vi "qEAX.vi"(0 "System no.":i32=1 min=1 max=4 step=1, 2 "Axes to query":string[](array[string]), 3 "All axes?":bool, 4 "Axis identifier?":bool=TRUE, 5 "error in":errorcluster) -> (14 "Axes enabled status":bool[](array[boolean]), 19 "error out":errorcluster)   [LabVIEW 2026]
doc: "GCS 3.0\n=====\n\nEAX? (Get Axis Activation State)\n\nDescription\nQueries the activation state of the axes.\nThe activation state of an axis corresponds to the switch-on state of its drive.\n\nFormat\nEAX?[ <AxisID>]\n\nArguments\nEAX? without arguments queries all axes of the controller.\n<AxisID>\nAn axis of the controller\nThe available axes can be queried with USG? SYS.\nPossible values: Alias of the axis\n\nResponse\n{<AxisID>\"=\"<ActivationState>LF}\n<ActivationState>\nActivation state of the axis\nCorresponds to the switch-on state of the drive of the axis\nPossible values:\n0 = Axis deactivated = Drive switched off\n1 = Axis activated = Drive switched on\n\nExample\n>>eax?\n<<AXIS_1=0\n<<AXIS_2=0\n>>eax axis_1 1\n>>eax?\n<<AXIS_1=1\n<<AXIS_2=0\n\nNotes\nMotion of the axis is only possible if the axis is activated with EAX. For further details, \nsee \"Drive State Machine\". \nThe activation state of the axes is set with the EAX command.\nIf a motion error occurs, the axis is automatically deactivated on the transition from the Fault \nreaction active state to the Fault state.\nThe activation state is also displayed in the status register of the axis, which can be \nqueried with the STV? command. \n\nUser command level\nUSR\n\n\nGCS 2.0\n=====\n\nReturns enabled status of queried axes.\n\nAll systems: If All axes? = TRUE, then Axis identifier? can be FALSE"
panel:
  # "EAX? (Get Axis Activation State)\n\nQueries the activation state of the axes.\nThe activation state of an axis corresponds to the switch-on state of its drive."
  # "Query"
  # "If all axes: use"
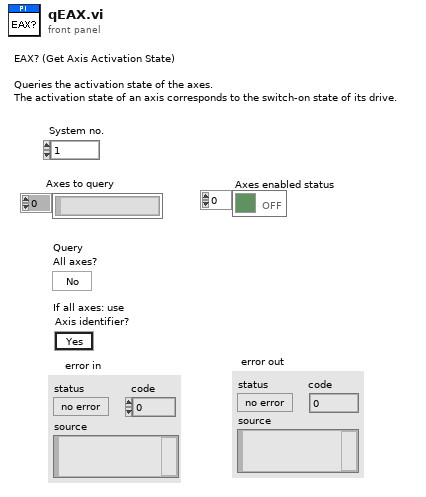
[diagram p1: front panel]
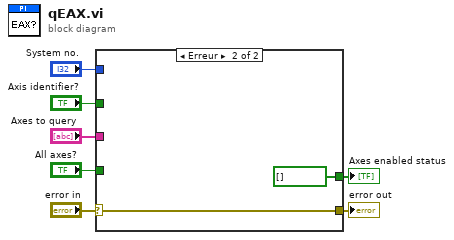
[diagram p0: block diagram]
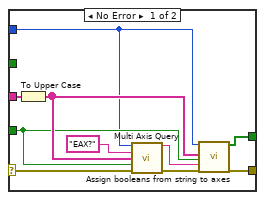
[diagram p2: hidden frame]
diagram:
  n1 = case shown="Erreur" "error in" {
    selector: "error in" -> [w16 w19]
    tunnel: [w11 bool[] [] ("Booleans")] -> w2
    tunnel: "Axes to query" -> [w17 _]
    tunnel: [w13 w19] -> w3
    tunnel: "System no." -> [w8 _]
    tunnel: "All axes?" -> [w9 _]
    tunnel: "Axis identifier?" -> [_ _]
    frame No Error {
      n2 = To Upper Case(1:w17) -> (0:w12:string[])
      n3 = call "Multi Axis Query.vi"("System no."=w8, "Command"="EAX?", "Axis"=w12, "All axes?"=w9, "error in (no error)"=w16) -> ("Answer"=w10:string, "error out"=w14:errorcluster)  [unwired: 9 in]
      n4 = call "Assign booleans from string to axes.vi"("System no."=w8, "Queried axes"=w12, "All axes queried?"=w9, "Input String"=w10, "error in"=w14) -> ("Booleans"=w11:bool[], "error out"=w13:errorcluster)  [unwired: 13 in]
    }
    frame Error {
      (unwired) string[] [] ("Axes to query out")
    }
  }
  "error out" <- w3
  "Axes enabled status" <- w2
